vi "niDTS WLAN UTIL ModAcc Pilot Tracking.vi"(8 "error in (no error)":errorcluster, 10 "Parameters":T1={"Standard"=enum."802.11 n HT", "DSSS Data Rate (Mbps)"=enum."1", "OFDM Data Rate (Mbps)"=enum."54", "MCS Index"=7, "N spatial streams"=1, "Chains"=[TRUE, FALSE, FALSE, FALSE], "BandWidth (Hz)"=enum."20 MHz", "Channel"=1, "Gard Interval"=enum."SHORT", "FEC Coding"=enum."LDPC", "Dut Tx Power"=0.0, "16 symbols"=TRUE, "payload length bytes"=1500, "idle interval"=0.0001, "External Attenuation"=[0.0, 0.0, 0.0, 0.0], "Acquisition Parameters "={"Acquisition Length Mode"=enum."MANUAL", "Acquisition Length (s)"=0.00015, "Auto Level"=FALSE}, "TXP Measurement Parameters"={"TXP Power Enable"=FALSE, "TXP Averages"=3}, "ModAcc Measurement Paramaters"={"ModAcc Enable"=FALSE, "Header Detection"=enum."FIRST", "Averages"=3, "Amplitude Tracking"=FALSE, "Channel Tracking"=FALSE, "Time Tracking"=FALSE, "Phase Tracking"=enum."NONE", "Clock Offset Est"=FALSE, "Impairments Est"=FALSE, "CFO Estimation"=enum."PAMBLE"}, "ModAcc DSSS Paramaters"={"DC Offset Compensation"=TRUE, "Equalization"=FALSE, "Phase Tracking"=FALSE, "Chip Start Location"=0, "Max Chips Used"=1, "Pulse Shaping FilterType"=enum."NONE", "Pulse Shaping Filter Coefficient"=1000.0}, "SEM Measurement Parameters"={"SEM Enable"=FALSE, "SEM Averages"=3, "Auto Span Enable"=TRUE, "Frequency Span (Hz)"=0.0, "Measurement Type"=enum."Standard", "Mask Frequencies (Hz)"=[], "Mask Power Offsets (dB)"=[]}, "OBW Measurement Parameters"={"OBW Enable"=FALSE, "OBW Averages"=3}, "DSSS Power Ramp"={"Power Ramp Enable"=FALSE, "Averages"=3, "Thresholds"={"Up Low (%)"=10.0, "Down Low (%)"=10.0, "Up High (%)"=90.0, "Down High (%)"=90.0}}, "Enable Traces"=FALSE} {"DSSS Power Ramp"."Thresholds"."Down High (%)" min=0.0 max=100.0 step=1.0; "DSSS Power Ramp"."Thresholds"."Up High (%)" min=0.0 max=100.0 step=1.0; "DSSS Power Ramp"."Thresholds"."Down Low (%)" min=0.0 max=100.0 step=1.0; "DSSS Power Ramp"."Thresholds"."Up Low (%)" min=0.0 max=100.0 step=1.0; "Acquisition Parameters"."Acquisition Length (s)" format="%#_6p"; "SEM Measurement Parameters"."Frequency Span (Hz)" format="%#_6p"; "idle interval" format="%_3p"}, 11 "Data Value Reference in":T16) -> (0 "error out":errorcluster, 3 "Data Value Reference out":T16)   [LabVIEW 2014, in "niDTS WLAN.lvlib"]
uses:
  niDTS WLAN.lvlib
  RiviInstDriver/niRfsaWlan/Includes/niRfsaWlan INC Handle.ctl
  RiviInstDriver/niRfsaWlan/Objects/niRfsaWlan.lvclass
  Tests/Tx Test/Includes/niDTS WLAN Tx Test INC Parameters.ctl
  Includes/niDTS WLAN INC Standard.ctl
  Includes/niDTS WLAN INC DSSS Data Rate.ctl
  Includes/niDTS WLAN INC OFDM Data Rate.ctl
  Includes/niDTS WLAN INC CH BW.ctl
  Includes/niDTS WLAN INC GI.ctl
  Includes/niDTS WLAN INC FEC Coding.ctl
  Includes/niDTS WLAN DUT INC Acquisition Parameters.ctl
  Includes/niDTS WLAN INC TXP Measurement Parameters.ctl
  Includes/niDTS WLAN INC ModAcc Measurement Parameters.ctl
  Includes/niDTS WLAN INC DSSS ModAcc Measurement Parameters.ctl
  Includes/niDTS WLAN INC Pulse Shaping Filter Type.ctl
  Includes/niDTS WLAN INC SEM Measurement Parameters.ctl
  Includes/niDTS WLAN INC OBW Measurement Parameters.ctl
  Includes/niDTS WLAN INC DSSS Power Ramp Parameters.ctl
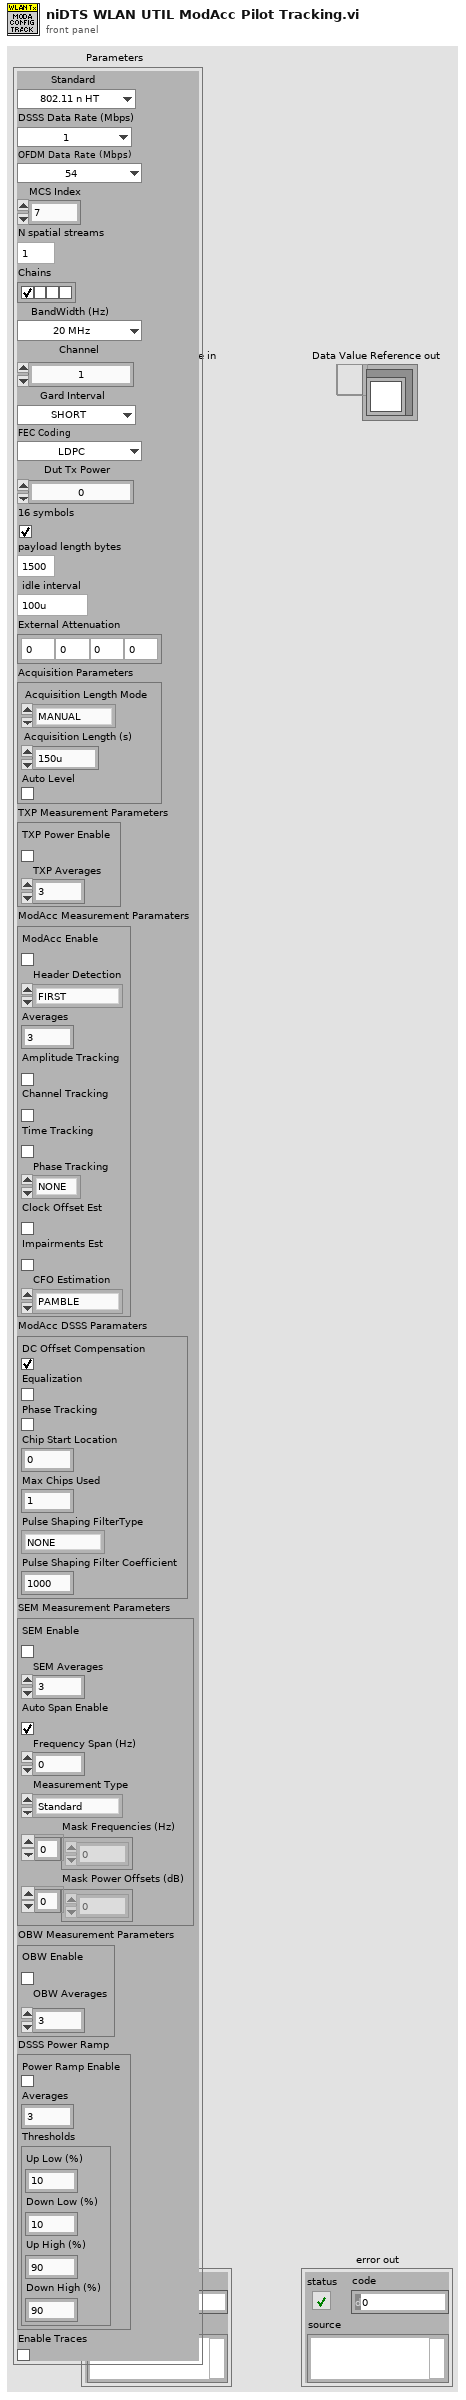
[diagram p1: front panel]
types:
  T1 = typedef "niDTS WLAN.lvlib/niDTS WLAN Tx Test INC Parameters.ctl" = cluster{"Standard":T2, "DSSS Data Rate (Mbps)":T3, "OFDM Data Rate (Mbps)":T4, "MCS Index":i32, "N spatial streams":i32, "Chains":bool[], "BandWidth (Hz)":T5, "Channel":i32, "Gard Interval":T6, "FEC Coding":T7, "Dut Tx Power":dbl, "16 symbols":bool, "payload length bytes":i32, "idle interval":dbl, "External Attenuation":dbl[], "Acquisition Parameters ":T8, "TXP Measurement Parameters":T9, "ModAcc Measurement Paramaters":T10, "ModAcc DSSS Paramaters":T11, "SEM Measurement Parameters":T13, "OBW Measurement Parameters":T14, "DSSS Power Ramp":T15, "Enable Traces":bool}
  T2 = typedef "niDTS WLAN.lvlib/niDTS WLAN INC Standard.ctl" = enum16{"802.11 b DSSS", "802.11 a/g OFDM", "802.11 n HT", "802.11 ac VHT"}
  T3 = typedef "niDTS WLAN.lvlib/niDTS WLAN INC DSSS Data Rate.ctl" = enum16{"1", "2", "5.5", "11"}
  T4 = typedef "niDTS WLAN.lvlib/niDTS WLAN INC OFDM Data Rate.ctl" = enum16{"6", "9", "12", "18", "24", "36", "48", "54"}
  T5 = typedef "niDTS WLAN.lvlib/niDTS WLAN INC CH BW.ctl" = enum16{"20 MHz", "40 MHz", "80 MHz", "160 MHz"}
  T6 = typedef "niDTS WLAN.lvlib/niDTS WLAN INC GI.ctl" = enum16{"LONG", "SHORT"}
  T7 = typedef "niDTS WLAN.lvlib/niDTS WLAN INC FEC Coding.ctl" = enum16{"BCC", "LDPC"}
  T8 = typedef "niDTS WLAN.lvlib/niDTS WLAN DUT INC Acquisition Parameters.ctl" = cluster{"Acquisition Length Mode":enum16{"AUTO", "MANUAL"}, "Acquisition Length (s)":dbl, "Auto Level":bool}
  T9 = typedef "niDTS WLAN.lvlib/niDTS WLAN INC TXP Measurement Parameters.ctl" = cluster{"TXP Power Enable":bool, "TXP Averages":i32}
  T10 = typedef "niDTS WLAN.lvlib/niDTS WLAN INC ModAcc Measurement Parameters.ctl" = cluster{"ModAcc Enable":bool, "Header Detection":enum16{"MANUAL", "FIRST", "ALL"}, "Averages":i32, "Amplitude Tracking":bool, "Channel Tracking":bool, "Time Tracking":bool, "Phase Tracking":enum16{"NONE", "STANDARD", "CSF", "INSTANT"}, "Clock Offset Est":bool, "Impairments Est":bool, "CFO Estimation":enum16{"PAMBLE", "PDATA"}}
  T11 = typedef "niDTS WLAN.lvlib/niDTS WLAN INC DSSS ModAcc Measurement Parameters.ctl" = cluster{"DC Offset Compensation":bool, "Equalization":bool, "Phase Tracking":bool, "Chip Start Location":i16, "Max Chips Used":i16, "Pulse Shaping FilterType":T12, "Pulse Shaping Filter Coefficient":dbl}
  T12 = typedef "niDTS WLAN.lvlib/niDTS WLAN INC Pulse Shaping Filter Type.ctl" = enum16{"NONE", "RCOSINE", "RRCOSINE", "GAUSSIAN"}
  T13 = typedef "niDTS WLAN.lvlib/niDTS WLAN INC SEM Measurement Parameters.ctl" = cluster{"SEM Enable":bool, "SEM Averages":i32, "Auto Span Enable":bool, "Frequency Span (Hz)":dbl, "Measurement Type":enum16{"Standard", "Legacy", "Custom"}, "Mask Frequencies (Hz)":dbl[], "Mask Power Offsets (dB)":dbl[]}
  T14 = typedef "niDTS WLAN.lvlib/niDTS WLAN INC OBW Measurement Parameters.ctl" = cluster{"OBW Enable":bool, "OBW Averages":i32}
  T15 = typedef "niDTS WLAN.lvlib/niDTS WLAN INC DSSS Power Ramp Parameters.ctl" = cluster{"Power Ramp Enable":bool, "Averages":i32, "Thresholds":cluster{"Up Low (%)":dbl, "Down Low (%)":dbl, "Up High (%)":dbl, "Down High (%)":dbl}}
  T16 = typedef "niRfsaWlan.lvclass/niRfsaWlan INC Handle.ctl" = refnum<data-value>
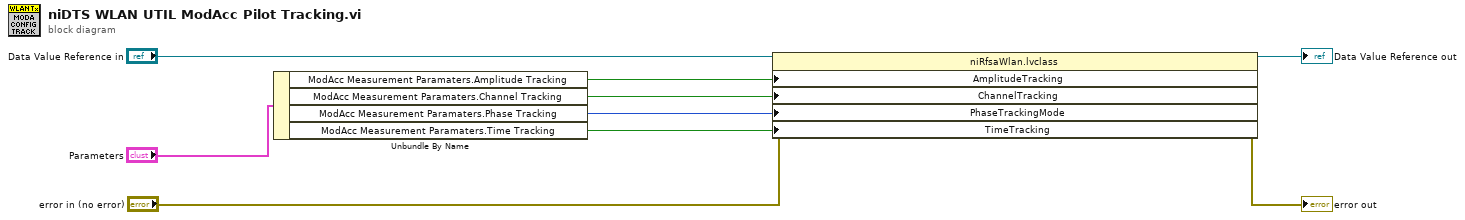
[diagram p0: block diagram]
diagram:
  n1 = Unbundle By Name("Parameters") -> ("ModAcc Measurement Paramaters.Amplitude Tracking"=w9:bool, "ModAcc Measurement Paramaters.Channel Tracking"=w8:bool, "ModAcc Measurement Paramaters.Phase Tracking"=w7:enum16{"NONE", "STANDARD", "CSF", "INSTANT"}, "ModAcc Measurement Paramaters.Time Tracking"=w6:bool)
  n2 = property class="niRfsaWlan.lvclass"(reference="Data Value Reference in", error in="error in (no error)", "AmplitudeTracking"=w9, "ChannelTracking"=w8, "PhaseTrackingMode"=w7, "TimeTracking"=w6) -> (reference out=→"Data Value Reference out":T16, error out=→"error out":errorcluster)
